vi "Close.vi"(8 "error in (no error)":errorcluster, 11 "TXT_Writer in":refnum<class "TXT_Writer.lvclass">) -> (0 "error out":errorcluster, 3 "TXT_Writer out":refnum<class "TXT_Writer.lvclass">)   [LabVIEW 2024, in "Data.lvlib" / "TXT_Writer.lvclass"]
uses:
  TXT_Writer.lvclass
  TXT_Writer.lvclass/TXT_Writer.ctl
  Data/DataWriter/DataWriter.lvclass
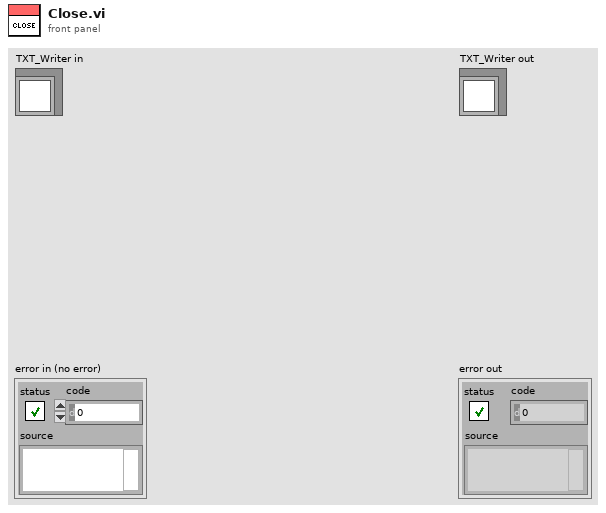
[diagram p1: front panel]
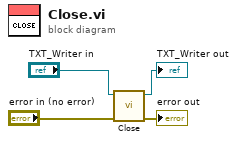
[diagram p0: block diagram]
diagram:
  n1 = call-parent "Close.vi"("error in (no error)"="error in (no error)", "DataWriter in"="TXT_Writer in") -> ("error out"=→"error out":errorcluster, "DataWriter out"=→"TXT_Writer out":refnum<class "TXT_Writer.lvclass">)  [unwired: 8 in]
